vi "Rearrange Controls.vi"(8 "error in":errorcluster {"code" format="%.0x"}, 10 "controls references":refnum<vi>[][](array[refnum])) -> (0 "error out":errorcluster {"code" format="%.0x"}, 2 "controls references out":refnum<vi>[][](array[refnum]), 4 "panel width":i16, 6 "panel height":i16)   [LabVIEW 2018, in "NISAST VI Scripting.lvlib" / "VI.lvlib" / "Front Panel.lvlib"]
uses:
  Front Panel.lvlib
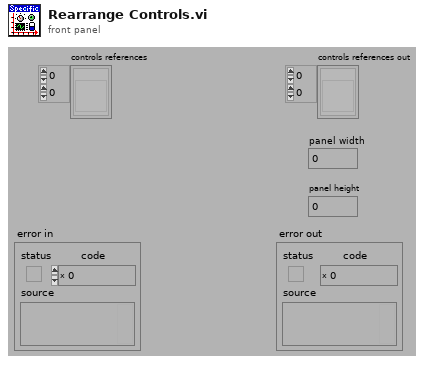
[diagram p1: front panel]
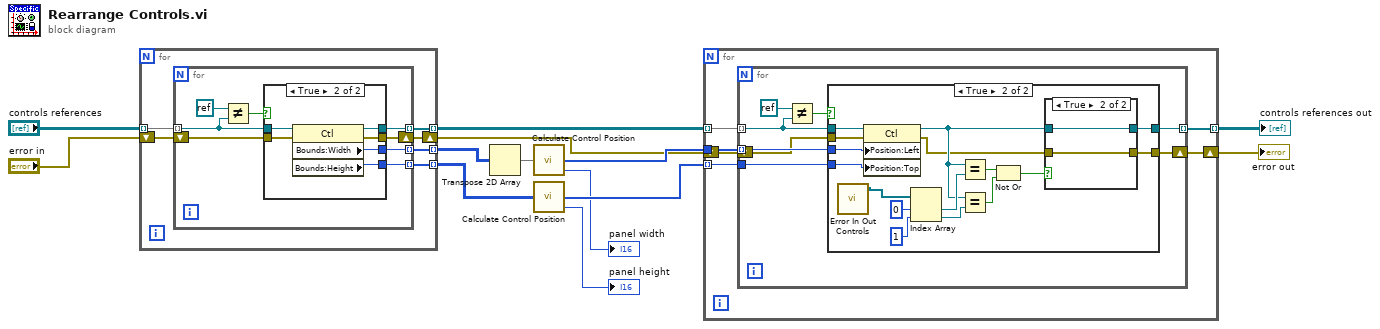
[diagram p0: block diagram]
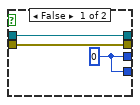
[diagram p4: hidden frame]
diagram:
  n1 = for {
    tunnel: "controls references" -> [w19] mode=indexing
    tunnel: [w18] -> w8 mode=indexing
    tunnel: [w17] -> w7 mode=indexing
    tunnel: [w16] -> w6 mode=indexing
    shift-right: [w15] -> w4
    shift-left: "error in" -> [w14]
    n2 = for {
      tunnel: w19 -> [w24] mode=indexing
      tunnel: [w27] -> w18 mode=indexing
      tunnel: [w26] -> w17 mode=indexing
      tunnel: [w25] -> w16 mode=indexing
      shift-right: [w21] -> w15
      shift-left: w14 -> [w20]
      n3 = Not Equal?(x=refnum<k0> refnum, y=w24) -> (x != y?=w22:bool)
      n4 = case shown="True" w22 {
        tunnel: [w29 w36] -> w27
        tunnel: [w29 w35] -> w26
        tunnel: [w30 w34] -> w25
        tunnel: w24 -> [w30 w33]
        tunnel: [w28 w32] -> w21
        tunnel: w20 -> [w28 w31]
        frame False {
          w29 = u32 0 ("Width")
        }
        frame True {
          n5 = property class="Ctl"(reference=w33, error in=w31) -> (reference out=w34:refnum<vi>, error out=w32:errorcluster, "Bounds:Width"=w36:u32, "Bounds:Height"=w35:u32)
        }
      }
    }
  }
  n6 = Transpose 2D Array(2D array=w8) -> (transposed array=w9:u32[][])
  n7 = call "Calculate Control Position.vi"("size array"=w9) -> ("position array"=w5:u32[], "sum value"=→"panel width":i16)  [unwired: 1 out]
  n8 = call "Calculate Control Position.vi"("size array"=w7) -> ("position array"=w3:u32[], "sum value"=→"panel height":i16)  [unwired: 1 out]
  n9 = for {
    tunnel: w6 -> [w42] mode=indexing
    tunnel: [w41] -> w12 mode=indexing
    tunnel: w5 -> [w40]
    shift-right: [w37] -> w10
    shift-left: w4 -> [w39]
    tunnel: w3 -> [w38] mode=indexing
    n10 = for {
      tunnel: w42 -> [w49] mode=indexing
      tunnel: [w50] -> w41 mode=indexing
      tunnel: w40 -> [w46] mode=indexing
      shift-right: [w43] -> w37
      shift-left: w39 -> [w44]
      tunnel: w38 -> [w45]
      n11 = Not Equal?(x=refnum<k0> refnum, y=w49) -> (x != y?=w47:bool)
      n12 = case shown="True" w47 {
        tunnel: [w52 w57] -> w50
        tunnel: w49 -> [w52 w68]
        tunnel: w46 -> [_ w67]
        tunnel: w45 -> [_ w66]
        tunnel: w44 -> [w51 w65]
        tunnel: [w51 w56] -> w43
        frame False {
        }
        frame True {
          n13 = call "Error In Out Controls.vi"() -> ("error in/out control out"=w53:refnum<vi>[])  [unwired: 2 in, 9 out]
          n14 = property class="Ctl"(reference=w68, error in=w65, "Position:Left"=w67, "Position:Top"=w66) -> (reference out=w58:refnum<vi>, error out=w55:errorcluster)
          n15 = Index Array(array=w53, index #1=0 ("index"), index #2=1 ("index")) -> (element #1=w62:refnum<vi>, element #2=w61:refnum<vi>)
          n16 = Equal?(x=w58, y=w62) -> (x = y?=w60:bool)
          n17 = Equal?(x=w58, y=w61) -> (x = y?=w59:bool)
          n18 = Not Or(1:w59, 2:w60) -> (0:w54:bool)
          n19 = case shown="True" w54 {
            tunnel: w58 -> [w70 w72]
            tunnel: [w70 w72] -> w57
            tunnel: [w69 w71] -> w56
            tunnel: w55 -> [w69 w71]
            frame False {
            }
            frame True {
            }
          }
        }
      }
    }
  }
  "error out" <- w10
  "controls references out" <- w12
